vi "CloseProgressBar.vi"(1 "error in":errorcluster, 2 "reference in":refnum<vi>) -> (0 "error out":errorcluster)   [LabVIEW 2018]
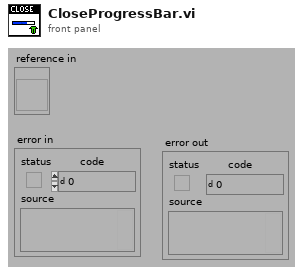
[diagram p1: front panel]
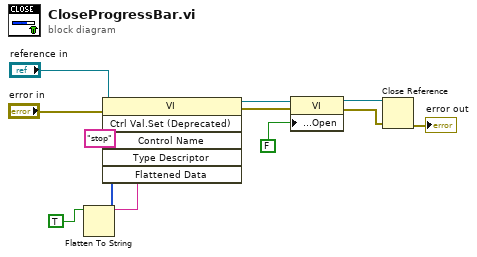
[diagram p0: block diagram]
diagram:
  n1 = Flatten To String(anything=TRUE) -> (data string=w10:string, type string=w9:i16[])  [unwired: 3 in, 1 out]
  n2 = invoke class="VI" method="Ctrl Val.Set (Deprecated)"(reference="reference in", error in="error in", "Control Name"="stop", "Type Descriptor"=w9, "Flattened Data"=w10) -> (reference out=w2:refnum<vi>, error out=w1:errorcluster)  [unwired: 1 in, 4 out]
  n3 = property class="VI"(reference=w2, error in=w1, "Front Panel Window:Open"=FALSE) -> (reference out=w3:refnum<vi>, error out=w4:errorcluster)
  n4 = Close Reference(reference=w3, error in (no error)=w4) -> (error out=→"error out":errorcluster)
